vi "rtout_controlTriggerConfig.vi"(0 "connection ID":refnum<k5>, 1 "axis in":i32, 2 "higher":i32, 3 "lower":i32, 4 "epsilon":i32, 5 "error in":errorcluster, 6 "Set":bool, 7 "polarity":i32) -> (13 "polarity out":i32, 14 "connection ID":refnum<k5>, 15 "axis out":i32, 16 "higher out":i32, 17 "lower out":i32, 18 "epsilon out":i32, 19 "error out":errorcluster)   [LabVIEW 2016]
doc: "By means of this VI the real time output trigger configuration is retrieved or set."
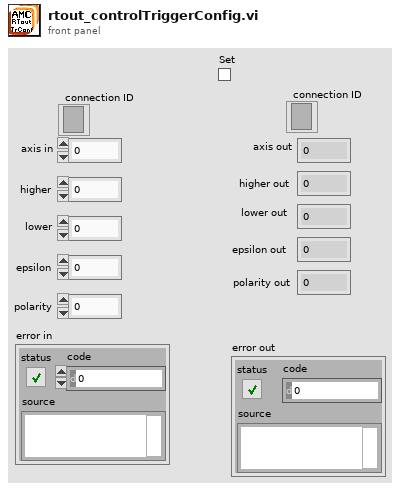
[diagram p1: front panel]
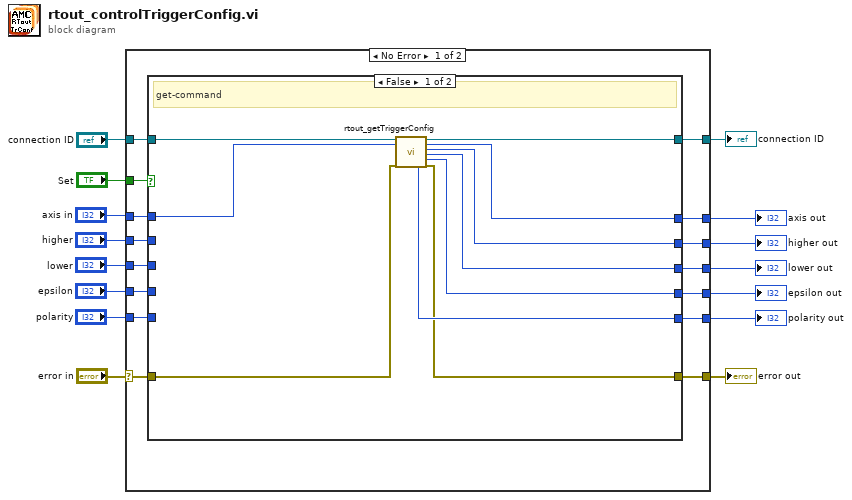
[diagram p0: block diagram]
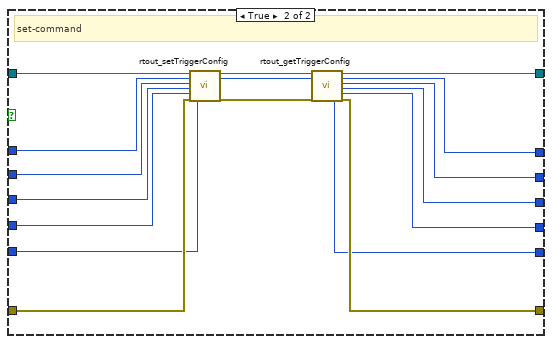
[diagram p2: hidden frame]
diagram:
  n1 = case shown="No Error" "error in" {
    selector: "error in" -> [w26 w64]
    tunnel: "axis in" -> [w30 w62]
    tunnel: [w24 w64] -> w14
    tunnel: "higher" -> [w28 w63]
    tunnel: [w25 w63] -> w9
    tunnel: "Set" -> [w27 _]
    tunnel: [w23 w58] -> w12
    tunnel: "connection ID" -> [w29 w58]
    tunnel: [w18 w62] -> w7
    tunnel: "lower" -> [w20 w61]
    tunnel: "epsilon" -> [w21 w60]
    tunnel: [w22 w60] -> w4
    tunnel: [w17 w61] -> w6
    tunnel: "polarity" -> [w19 w59]
    tunnel: [w16 w59] -> w1
    frame No Error {
      n2 = case shown="False" w27 {
        tunnel: w29 -> [w40 w57]
        tunnel: w30 -> [w38 w51]
        tunnel: w28 -> [_ w50]
        tunnel: w26 -> [w37 w52]
        tunnel: [w32 w44] -> w25
        tunnel: [w35 w53] -> w24
        tunnel: [w39 w55] -> w23
        tunnel: w20 -> [_ w49]
        tunnel: w21 -> [_ w48]
        tunnel: [w34 w42] -> w22
        tunnel: w19 -> [_ w47]
        tunnel: [w31 w45] -> w18
        tunnel: [w33 w43] -> w17
        tunnel: [w36 w41] -> w16
        frame False {
          # "get-command"
          n3 = call "rtout_getTriggerConfig.vi"("connection ID"=w40, "axis"=w38, "error in"=w37) -> ("polarity"=w36:i32, "connection ID"=w39:refnum<k5>, "axis_out"=w31:i32, "higher"=w32:i32, "lower"=w33:i32, "epsilon"=w34:i32, "error out"=w35:errorcluster)  [unwired: 10 in]
        }
        frame True {
          # "set-command"
          n4 = call "rtout_setTriggerConfig.vi"("connection ID"=w57, "axis"=w51, "higher"=w50, "lower"=w49, "epsilon"=w48, "error in"=w52, "polarity"=w47) -> ("connection ID"=w56:refnum<k5>, "axis_out"=w46:i32, "error out"=w54:errorcluster)  [unwired: 10 in]
          n5 = call "rtout_getTriggerConfig.vi"("connection ID"=w56, "axis"=w46, "error in"=w54) -> ("polarity"=w41:i32, "connection ID"=w55:refnum<k5>, "axis_out"=w45:i32, "higher"=w44:i32, "lower"=w43:i32, "epsilon"=w42:i32, "error out"=w53:errorcluster)  [unwired: 10 in]
        }
      }
    }
    frame Error {
    }
  }
  "error out" <- w14
  "axis out" <- w7
  "higher out" <- w9
  "connection ID" <- w12
  "lower out" <- w6
  "epsilon out" <- w4
  "polarity out" <- w1
